vi "QueryAxisPosition.vi"(8 "error in (no error)":errorcluster, 11 "Picomoto8742ControllerClass in":refnum<class "Picomoto8742ControllerClass.lvclass">) -> (0 "error out":errorcluster, 3 "Picomoto8742ControllerClass out":refnum<class "Picomoto8742ControllerClass.lvclass">)   [LabVIEW 2013, in "Picomoto8742ControllerClass.lvclass"]
doc: "Query the position relative to the active axis, from the physical device"
uses:
  Picomoto8742ControllerClass.lvclass
  Picomoto8742ControllerClass.lvclass/Picomoto8742ControllerClass.ctl
  Picomotor8742Axis.lvclass
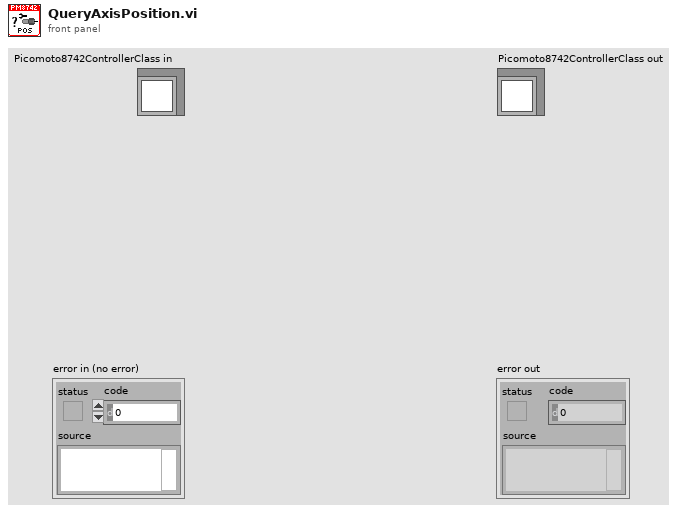
[diagram p1: front panel]
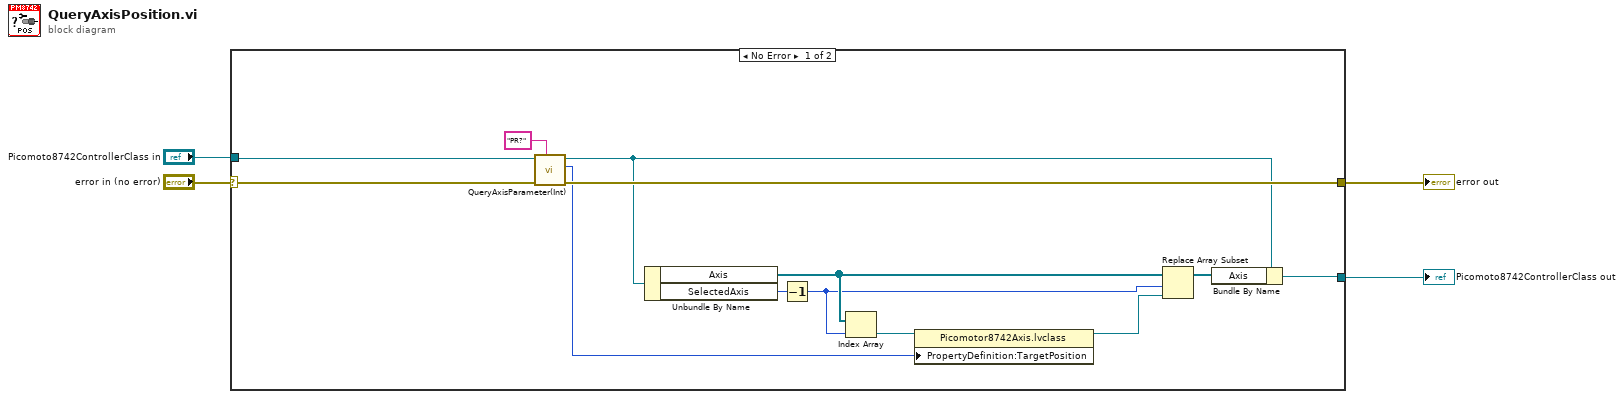
[diagram p0: block diagram]
diagram:
  n1 = case shown="No Error" "error in (no error)" {
    selector: "error in (no error)" -> [w6 w19]
    tunnel: [w17 w19] -> w3
    tunnel: [w14 w18] -> w1
    tunnel: "Picomoto8742ControllerClass in" -> [w7 w18]
    frame No Error {
      n2 = call-dynamic "QueryAxisParameter(Int).vi"("Cmd"="PR?" ("string"), "error in (no error)"=w6, "Picomoto8742ControllerClass in"=w7) -> ("error out"=w17:errorcluster, "ValueOut"=w5:i32, "Picomoto8742ControllerClass Out"=w9:refnum<class "Picomoto8742ControllerClass.lvclass">)  [unwired: 6 in]
      n3 = Unbundle By Name(w9) -> ("Axis"=w12:refnum<class "Picomotor8742Axis.lvclass">[], "SelectedAxis"=w11:u32)
      n4 = Decrement(x=w11) -> (x-1=w8:u32)
      n5 = Index Array(array=w12, index=w8) -> (element=w10:refnum<class "Picomotor8742Axis.lvclass">)
      n6 = property class="Picomotor8742Axis.lvclass"(reference=w10, "PropertyDefinition:TargetPosition"=w5) -> (reference out=w16:refnum<class "Picomotor8742Axis.lvclass">)  [unwired: 1 in, 1 out]
      n7 = Replace Array Subset(array=w12, new element=w16, index=w8) -> (w15:refnum<class "Picomotor8742Axis.lvclass">[])
      n8 = Bundle By Name(cluster=w9, "Axis"=w15) -> (w14:refnum<class "Picomoto8742ControllerClass.lvclass">)
    }
    frame Error {
    }
  }
  "error out" <- w3
  "Picomoto8742ControllerClass out" <- w1
